vi "qSSN.vi"(0 "System no.":i32=1 min=1 max=4 step=1, 2 "Channel name":string=" ", 4 "With channel ID?":bool, 5 "error in":errorcluster) -> (14 "Serial number":string, 19 "error out":errorcluster)   [LabVIEW 2020]
doc: "Returns controller serial number. \n\nE-816: With channel ID = TRUE. This command cannot be issued to a slave.\n\nAll other systems: With channel ID = FALSE\n\nC-887, F-206, M-8X0: Only for GCS syntax version = GCS 2.0 or higher (check with CSV?.vi. If CSV?.vi is not supported, syntax version is GCS 1.0)."
panel:
  # "Returns controller serial number."
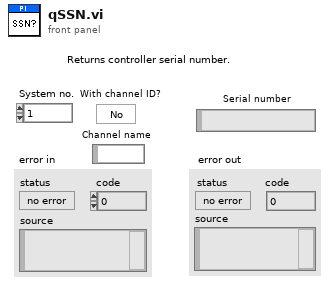
[diagram p1: front panel]
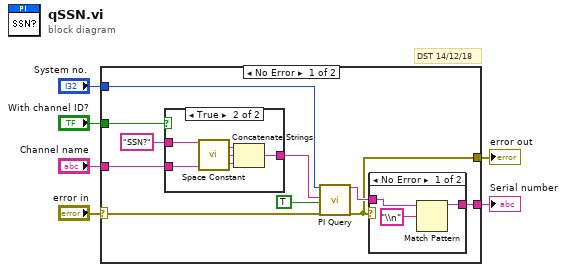
[diagram p0: block diagram]
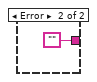
[diagram p3: hidden frame]
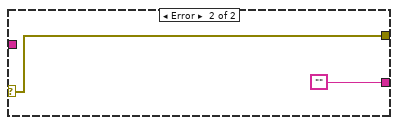
[diagram p4: hidden frame]
diagram:
  # "DST 14/12/18"
  n1 = case shown="No Error" "error in" {
    selector: "error in" -> [w7 w27]
    tunnel: "System no." -> [w15 _]
    tunnel: "With channel ID?" -> [w14 _]
    tunnel: [w11 ""] -> w4
    tunnel: "Channel name" -> [w10 _]
    tunnel: [w8 w27] -> w2
    frame No Error {
      n2 = case shown="True" w14 {
        tunnel: "SSN?" -> [w17 w20]
        tunnel: [w17 w19] -> w12
        tunnel: w10 -> [_ w18]
        frame False {
        }
        frame True {
          n3 = call <vilib>:"Space Constant.vi"() -> ("String"=w21:string)
          n4 = Concatenate Strings(w20, w21, w18) -> (w19:string)
        }
      }
      n5 = call "PI Query.vi"("System no."=w15, "String to send"=w12, "Attach termination char.?"=TRUE ("Attach Linefeed?"), "error in"=w7) -> ("String read"=w9:string, "error out"=w8:errorcluster)  [unwired: 3 in, 11 out]
      n6 = case shown="No Error" w8 {
        tunnel: w9 -> [w24 _]
        tunnel: [w22 "" ("String read")] -> w11
        frame No Error {
          n7 = Match Pattern(string=w24, regular expression="\\n") -> (before substring=w22:string)  [unwired: 4 out]
        }
        frame Error {
        }
      }
    }
    frame Error {
    }
  }
  "error out" <- w2
  "Serial number" <- w4
